vi "BadgeScan.vi"(8 "error in":errorcluster) -> (0 "error out":errorcluster)   [LabVIEW 2019]
uses:
  <vilib>/event_ctls.llb/eventvkey.ctl
panel:
  in  "Scan Badge to login":string
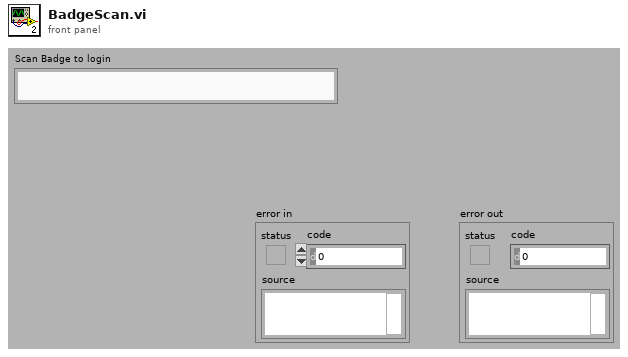
[diagram p1: front panel]
types:
  T1 = typedef "eventvkey.ctl" = enum16{"ASCII", "Enter", "Return", "Shift", "Ctrl", "Alt", "Cmd", "Opt", "Caps", "NumLock", "Clear", "Break", "Up", "Down", "Left", "Right", "Insert", "Delete", "Home", "End", "PageUp", "PageDown", "Escape", "Help", "Pause", "ScrollLock", "F1", "F2", "F3", "F4", "F5", "F6", "F7", "F8", "F9", "F10", "F11", "F12", "F13", "F14", "F15", "F16", "F17", "F18", "F19", "F20", "F21", "F22", "F23", "F24", "Play", "VolumeUp", "VolumeDown", "Mute", "Two Byte Char"}
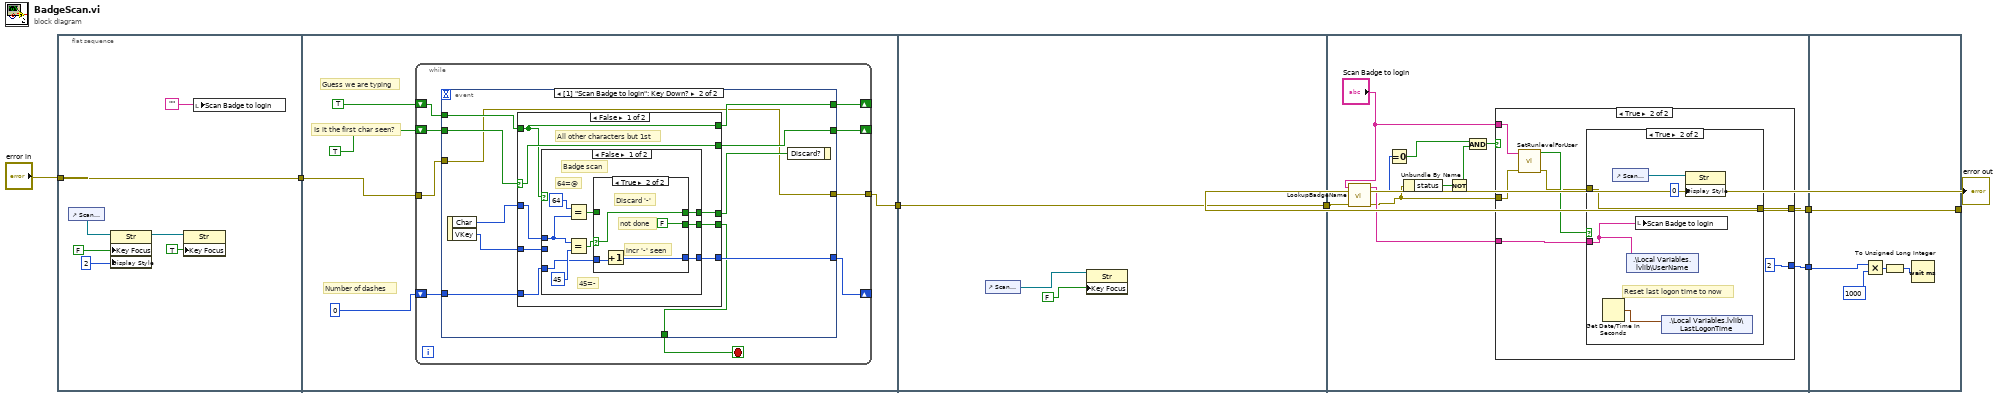
[diagram p0: block diagram]
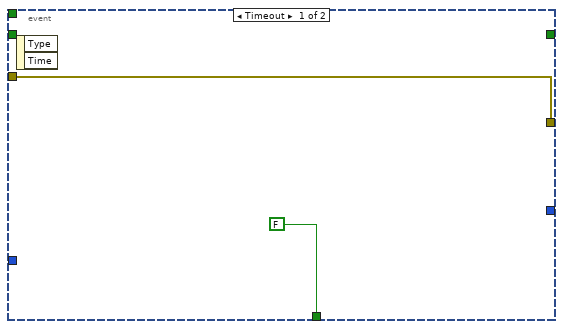
[diagram p2: hidden frame]
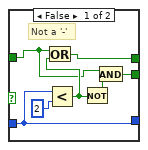
[diagram p3: hidden frame]
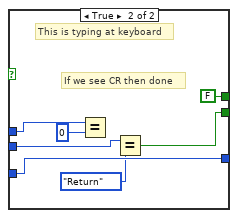
[diagram p4: hidden frame]
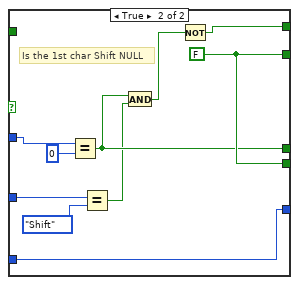
[diagram p5: hidden frame]
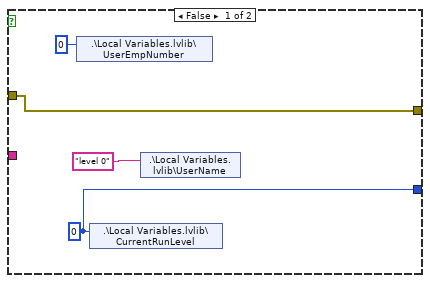
[diagram p6: hidden frame]
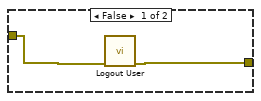
[diagram p7: hidden frame]
diagram:
  n1 = flat-sequence {
    tunnel: "error in" -> [w14]
    tunnel: [w14] -> w6
    tunnel: w6 -> [w19]
    tunnel: [w18] -> w2
    tunnel: w2 -> [w89]
    tunnel: [w89] -> w1
    tunnel: w1 -> [w98]
    tunnel: [w100] -> w4
    tunnel: [w96] -> w3
    tunnel: [w123] -> w5
    tunnel: w4 -> [w123]
    tunnel: w3 -> [w122]
    frame #0 {
      n2 = control-ref of="Scan Badge to login"() -> (w12:refnum<vi>)
      n3 = property class="Str"(reference=w12, "Key Focus"=FALSE, "Display Style"=u32 2) -> (reference out=w9:refnum<vi>)  [unwired: 1 in, 1 out]
      n4 = property class="Str"(reference=w9, "Key Focus"=TRUE) -> ()  [unwired: 1 in, 2 out]
      n5 = local write "Scan Badge to login"("") -> ()
    }
    frame #1 {
      # "Number of dashes"
      # "Is it the first char seen?"
      # "Guess we are typing"
      n6 = while {
        tunnel: w19 -> [w27]
        tunnel: [w26] -> w18
        shift-right: [w24] -> _
        shift-left: TRUE -> [w25]
        shift-right: [w22] -> _
        shift-left: TRUE -> [w23]
        shift-right: [w20] -> _
        shift-left: 0 -> [w21]
        stop <- w28 stop-if-true
        n7 = event shown="[1] \"Scan Badge to login\": Key Down?" {
          selector: _ -> [_ _]
          dyn-events: _ -> [_ _]
          timeout: _ -> [_ _]
          tunnel: [FALSE w33] -> w28
          tunnel: w27 -> [w29 w31]
          tunnel: [w29 w31] -> w26
          tunnel: w25 -> [_ w39]
          tunnel: [_ w38] -> w24
          tunnel: w23 -> [_ w41]
          tunnel: [_ w40] -> w22
          tunnel: w21 -> [_ w36]
          tunnel: [_ w34] -> w20
          event Timeout {
            n8 = event-data() -> ()  [unwired: 1 in, 2 out]
          }
          event "Scan Badge to login": Key Down? {
            n9 = event-data() -> ("Char"=w35:i16, "VKey"=w32:T1)  [unwired: 1 in]
            n10 = case shown="False" w41 {
              selector: w41 -> [w49 _]
              tunnel: [w49 w82] -> w40
              tunnel: w35 -> [w45 w86]
              tunnel: w39 -> [w48 _]
              tunnel: [w48 w83] -> w38
              tunnel: [w47 w79] -> w37
              tunnel: w36 -> [w46 w84]
              tunnel: [w44 w84] -> w34
              tunnel: [w43 w82] -> w33
              tunnel: w32 -> [w42 w81]
              frame False {
                # "All other characters but 1st"
                n11 = case shown="False" w48 {
                  tunnel: [w54 FALSE] -> w47
                  tunnel: w46 -> [w56 w76]
                  tunnel: w45 -> [w53 w75]
                  tunnel: [w55 w76] -> w44
                  tunnel: [w50 w71] -> w43
                  tunnel: w42 -> [_ w73]
                  frame False {
                    # "45=-"
                    # "64=@"
                    # "Badge scan"
                    n12 = Equal?(x=i16 64, y=w53) -> (x = y?=w51:bool)
                    n13 = Equal?(x=w53, y=i16 45) -> (x = y?=w57:bool)
                    n14 = case shown="True" w57 {
                      selector: w57 -> [_ w67]
                      tunnel: w56 -> [w63 w69]
                      tunnel: [w63 w68] -> w55
                      tunnel: [w65 w67] -> w54
                      tunnel: w51 -> [w60 _]
                      tunnel: [w59 FALSE] -> w50
                      frame False {
                        # "Not a '-'"
                        n15 = Less?(x=w63, y=2 ("x")) -> (x < y?=w62:bool)
                        n16 = Or(x=w60, y=w62) -> (x .or. y?=w65:bool)
                        n17 = Not(x=w62) -> (.not. x?=w61:bool)
                        n18 = And(x=w60, y=w61) -> (x .and. y?=w59:bool)
                      }
                      frame True {
                        # "not done"
                        # "incr '-' seen"
                        # "Discard '-'"
                        n19 = Increment(x=w69) -> (x+1=w68:i32)
                      }
                    }
                  }
                  frame True {
                    # "If we see CR then done"
                    # "This is typing at keyboard"
                    n20 = Equal?(x=w75, y=i16 0) -> ()  [unwired: 1 out]
                    n21 = Equal?(x=w73, y=eventvkey."Return" ("VKey")) -> (x = y?=w71:bool)
                  }
                }
              }
              frame True {
                w82 = FALSE
                # "Is the 1st char Shift NULL"
                n22 = Equal?(x=w86, y=i16 0) -> (x = y?=w79:bool)
                n23 = Equal?(x=w81, y=eventvkey."Shift") -> (x = y?=w78:bool)
                n24 = And(x=w79, y=w78) -> (x .and. y?=w77:bool)
                n25 = Not(x=w77) -> (.not. x?=w83:bool)
              }
            }
            n26 = event-data("Discard?"=w37) -> ()  [unwired: 1 in, 1 out]
          }
        }
      }
    }
    frame #2 {
      n27 = control-ref of="Scan Badge to login"() -> (w88:refnum<vi>)
      n28 = property class="Str"(reference=w88, "Key Focus"=FALSE) -> ()  [unwired: 1 in, 2 out]
    }
    frame #3 {
      n29 = call "LookupBadgeName.vi"("error in (no error)"=w98, "badgename"="Scan Badge to login") -> ("error out"=w94:errorcluster, "return type"=w95:u32, "fullname"=w99:string)  [unwired: 7 in]
      n30 = Equal To 0?(x=w95) -> (x = 0?=w91:bool)
      n31 = Unbundle By Name(w94) -> ("status"=w93:bool)
      n32 = Not(x=w93) -> (.not. x?=w90:bool)
      n33 = And(x=w91, y=w90) -> (x .and. y?=w92:bool)
      n34 = case shown="True" w92 {
        tunnel: w99 -> [_ w109]
        tunnel: w94 -> [w103 w111]
        tunnel: [w103 w105] -> w100
        tunnel: "Scan Badge to login" -> [_ w110]
        tunnel: [w101 2] -> w96
        frame False {
          w101 = 0 ("CurrentRunLevel")
          n35 = shared-variable ".\\Local Variables.lvlib\\UserEmpNumber"(0 ("UserEmpNumber")) -> ()  [unwired: 1 in, 1 out]
          n36 = shared-variable ".\\Local Variables.lvlib\\CurrentRunLevel"(w101) -> ()  [unwired: 1 in, 1 out]
          n37 = shared-variable ".\\Local Variables.lvlib\\UserName"("level 0" ("UserName")) -> ()  [unwired: 1 in, 1 out]
        }
        frame True {
          n38 = call "SetRunlevelForUser.vi"("error in (no error)"=w111, "LoginName"=w110) -> ("error out"=w106:errorcluster, "Logon Success"=w107:bool)  [unwired: 8 in]
          n39 = case shown="True" w107 {
            tunnel: w109 -> [_ w118]
            tunnel: w106 -> [w113 w116]
            tunnel: [w112 w116] -> w105
            frame False {
              n40 = call "Logout User.vi"("error in (no error)"=w113) -> ("error out"=w112:errorcluster)  [unwired: 10 in]
            }
            frame True {
              # "Reset last logon time to now"
              n41 = Get Date/Time In Seconds() -> (seconds since 1Jan1904=w117:timestamp)
              n42 = control-ref of="Scan Badge to login"() -> (w115:refnum<vi>)
              n43 = shared-variable ".\\Local Variables.lvlib\\UserName"(w118) -> ()  [unwired: 1 in, 1 out]
              n44 = local write "Scan Badge to login"(w118) -> ()
              n45 = shared-variable ".\\Local Variables.lvlib\\LastLogonTime"(w117) -> ()  [unwired: 1 in, 1 out]
              n46 = property class="Str"(reference=w115, "Display Style"=u32 0) -> ()  [unwired: 1 in, 2 out]
            }
          }
        }
      }
    }
    frame #4 {
      n47 = Multiply(x=w122, y=1000) -> (x*y=w120:i32)
      n48 = To Unsigned Long Integer(number=w120) -> (unsigned 32bit integer=w119:u32)
      n49 = Wait (ms)(milliseconds to wait=w119) -> ()  [unwired: 1 out]
    }
  }
  "error out" <- w5
